vi "DeviceWrite.vi"(4 "error in (no error)":errorcluster, 5 "Command":string, 6 "DeviceKey In":string, 7 "CmdLib In":refnum<k24>) -> (0 "error out":errorcluster, 2 "DeviceKey Out":string, 3 "CmdLib Out":refnum<k24>)   [LabVIEW 2013]
uses:
  C:/GEECS/Developers Version/builds/Device builds/Picomotor8742dotNet/CmdLib.dll
  CmdLib.dll
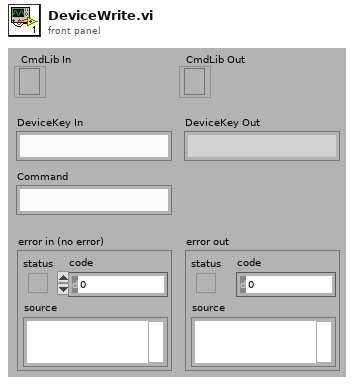
[diagram p1: front panel]
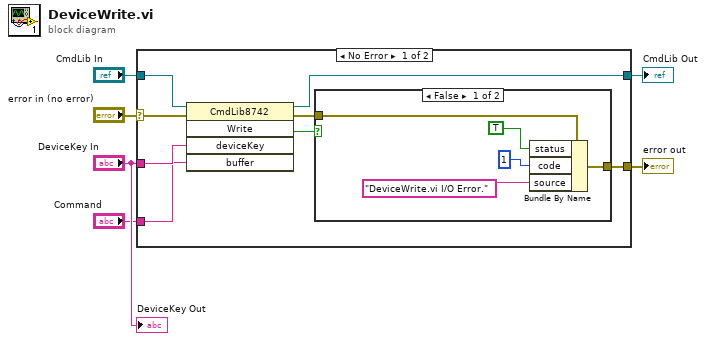
[diagram p0: block diagram]
diagram:
  n1 = case shown="No Error" "error in (no error)" {
    selector: "error in (no error)" -> [w11 w22]
    tunnel: "CmdLib In" -> [w14 w21]
    tunnel: [w13 w21] -> w5
    tunnel: "DeviceKey In" -> [w12 _]
    tunnel: [w8 w22] -> w2
    tunnel: "Command" -> [w7 _]
    frame No Error {
      n2 = invoke class="CmdLib8742" method="Write"(reference=w14, error in=w11, "deviceKey"=w12, "buffer"=w7) -> (reference out=w13:refnum<k24>, error out=w9:errorcluster, "Write"=w10:bool)  [unwired: 1 in, 2 out]
      n3 = case shown="False" w10 {
        tunnel: w9 -> [w17 w20]
        tunnel: [w16 w20] -> w8
        frame False {
          n4 = Bundle By Name(cluster=w17, "status"=TRUE, "code"=1, "source"="DeviceWrite.vi I/O Error.") -> (w16:errorcluster)
        }
        frame True {
        }
      }
    }
    frame Error {
    }
  }
  "CmdLib Out" <- w5
  "error out" <- w2
  "DeviceKey Out" <- "DeviceKey In"
